vi "ST example communication.vi"() -> ()   [LabVIEW 2009]
panel:
  out "Result Code":i32
  in  "String to send":string="PURGE"
  out "Output Valid":bool
  out "String Heard":string
  in  "Time Out":i32=10000
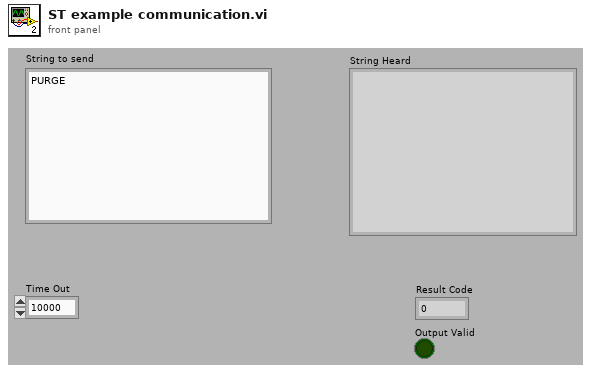
[diagram p1: front panel]
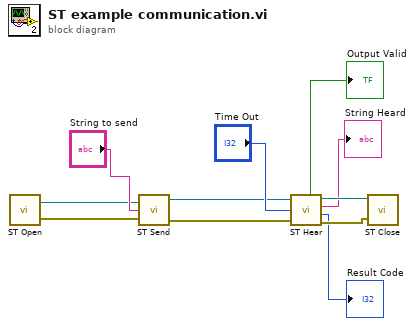
[diagram p0: block diagram]
diagram:
  n1 = call "ST Open.vi"() -> ("VISA resource name out"=w2:refnum<visa-resource-name>, "error out"=w3:errorcluster)  [unwired: 1 in]
  n2 = call "ST Send.vi"("error in (no error)"=w3, "String"="String to send", "VISA resource name"=w2) -> ("error out"=w4:errorcluster, "VISA resource name out"=w5:refnum<visa-resource-name>)  [unwired: 1 out]
  n3 = call "ST Hear.vi"("VISA resource name"=w5, "Time Out"="Time Out", "error in (no error)"=w4) -> ("VISA resource name out"=w11:refnum<visa-resource-name>, "String Received"=→"String Heard":string, "Result Code"=→"Result Code":i32, "error out"=w10:errorcluster, "Ready and OK"=→"Output Valid":bool)
  n4 = call "ST Close.vi"("error in (no error)"=w10, "VISA resource name"=w11) -> ()
